vi "ReadMercuryLegacy.vi"() -> ()   [LabVIEW 2014]
panel:
  out "Pool Bite":dbl
  in  "error in (no error)":errorcluster
  out "error out":errorcluster
  out "String 4":string
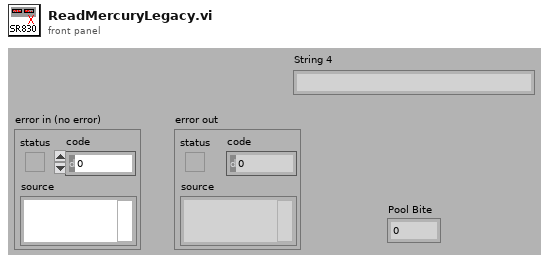
[diagram p1: front panel]
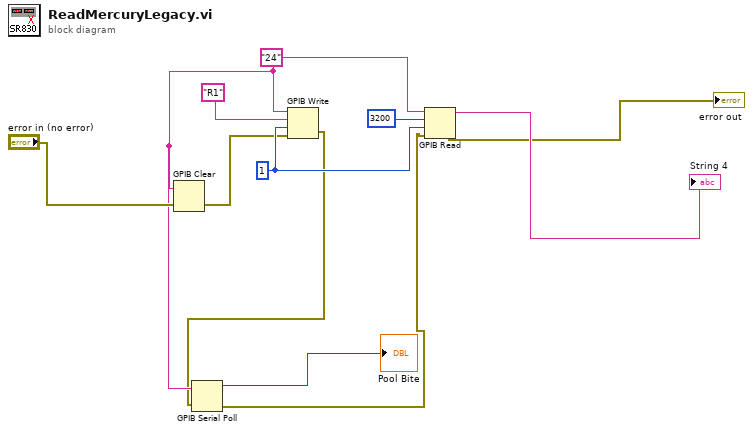
[diagram p0: block diagram]
diagram:
  w7 = 1
  w5 = "24"
  n1 = GPIB Clear(2:"error in (no error)", 3:w5) -> (0:w3:errorcluster)  [unwired: 1 out]
  n2 = GPIB Write(0:w5, 1:"R1", 2:w7, 3:w3) -> (6:w2:errorcluster)  [unwired: 1 in, 1 out]
  n3 = GPIB Serial Poll(0:w5, 1:w2) -> (2:→"Pool Bite":i16, 4:w1:errorcluster)  [unwired: 1 out]
  n4 = GPIB Read(0:w5, 1:3200, 2:w7, 3:w1) -> (5:→"String 4":string, 7:→"error out":errorcluster)  [unwired: 1 in, 1 out]
